vi "Anritsu VNA Get Stimulus.vi"(7 "Anritsu VNA":T1, 8 "error in (no error)":errorcluster, 9 "Channel":i8=1 min=1 max=99 step=1, 11 "VISA Resource Name":refnum<visa-resource-name>) -> (0 "error out":errorcluster, 2 "SP Stimulus":T2={"Use Instrument Settings"=FALSE, "Blank Frequencies"=FALSE, "Sweep Type"=enum."Linear", "Sweep"={"Fstart"=500.0, "Fstop"=1500.0, "Units"=enum."MHz", "Points"=201}, "Power (dBm)"=999.0, "IFBW (Hz)"=-1.0, "Sweep Time (s)"=-1.0, "Calibration"={"State"=FALSE, "String"=""}} {"Sweep Time (s)" format="%.3g"}, 3 "dup VISA Resource Name":refnum<visa-resource-name>)   [LabVIEW 2011]
uses:
  tests/S Parameter/TypeDefs/SP Stimulus Parameters.ctl
  tests/S Parameter/TypeDefs/SP Frequency Units.ctl
  tests/S Parameter/TypeDefs/SP Calibration State.ctl
  TypeDefs/Anritsu VNA Instrument Info.ctl
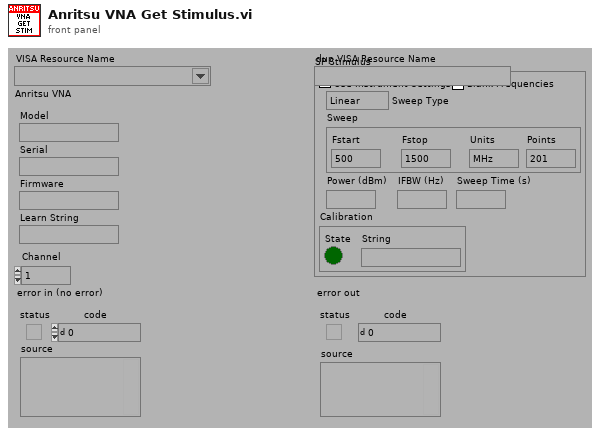
[diagram p1: front panel]
types:
  T1 = typedef "Anritsu VNA Instrument Info.ctl" = cluster{"Model":string, "Serial":string, "Firmware":string, "Learn String":string}
  T2 = typedef "SP Stimulus Parameters.ctl" = cluster{"Use Instrument Settings":bool, "Blank Frequencies":bool, "Sweep Type":enum32{"Linear", "Logarithmic", "List", "Power", "CW"}, "Sweep":cluster{"Fstart":dbl, "Fstop":dbl, "Units":T3, "Points":i32}, "Power (dBm)":dbl, "IFBW (Hz)":dbl, "Sweep Time (s)":dbl, "Calibration":T4}
  T3 = typedef "SP Frequency Units.ctl" = enum16{"Hz", "kHz", "MHz", "GHz", "Points"}
  T4 = typedef "SP Calibration State.ctl" = cluster{"State":bool, "String":string}
  T5 = typedef "Anritsu VNA Sweep Type.ctl" = enum32{"Linear Sweep", "Frequency Sweep", "Power Sweep", "CW Time Sweep", "Discrete Fill", "Time Domain", "Logarithmic Sweep", "Segmented Sweep (Frequency)", "Segmented Sweep (Index)", "MFGC"}
  T6 = enum32{"Linear", "Logarithmic", "List", "Power", "CW"}
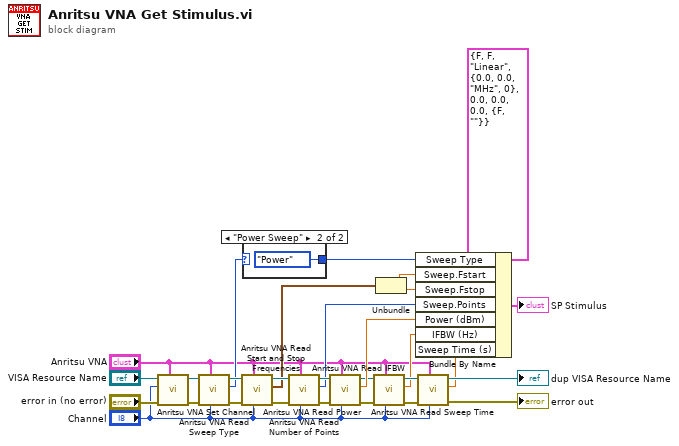
[diagram p0: block diagram]
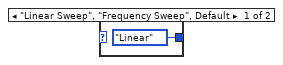
[diagram p2: hidden frame]
diagram:
  n1 = call "Anritsu VNA Set Channel.vi"("Anritsu VNA"="Anritsu VNA", "error in (no error)"="error in (no error)", "Channel"="Channel", "VISA Resource Name"="VISA Resource Name") -> ("error out"=w3:errorcluster, "dup VISA Resource Name"=w4:refnum<visa-resource-name>)  [unwired: 6 out]
  n2 = call "Anritsu VNA Read Sweep Type.vi"("Channel"="Channel", "Anritsu VNA"="Anritsu VNA", "error in (no error)"=w3, "VISA Resource Name"=w4) -> ("error out"=w27:errorcluster, "Sweep Type"=w20:T5, "dup VISA Resource Name"=w26:refnum<visa-resource-name>)  [unwired: 5 out]
  n3 = call "Anritsu VNA Read Start and Stop Frequencies.vi"("Channel"="Channel", "Anritsu VNA"="Anritsu VNA", "error in (no error)"=w27, "VISA Resource Name"=w26) -> ("error out"=w25:errorcluster, "Start/Stop Freqs, MHz"=w8:cluster{"Fstart":dbl, "Fstop":dbl}, "dup VISA Resource Name"=w24:refnum<visa-resource-name>)  [unwired: 5 out]
  n4 = case shown="\"Power Sweep\"" w20 {
    tunnel: [T6."Linear" ("Sweep Type") T6."Power" ("Sweep Type")] -> w7
    frame "Linear Sweep", "Frequency Sweep", Default {
    }
    frame "Power Sweep" {
    }
  }
  n5 = call "Anritsu VNA Read Number of Points.vi"("Channel"="Channel", "Anritsu VNA"="Anritsu VNA", "error in (no error)"=w25, "VISA Resource Name"=w24) -> ("error out"=w22:errorcluster, "Number Points"=w11:i32, "dup VISA Resource Name"=w23:refnum<visa-resource-name>)  [unwired: 5 out]
  n6 = call "Anritsu VNA Read Power.vi"("Channel"="Channel", "Anritsu VNA"="Anritsu VNA", "error in (no error)"=w22, "VISA Resource Name"=w23) -> ("error out"=w14:errorcluster, "Source Power, dBm"=w28:dbl, "dup VISA Resource Name"=w19:refnum<visa-resource-name>)  [unwired: 5 out]
  n7 = call "Anritsu VNA Read IFBW.vi"("Channel"="Channel", "Anritsu VNA"="Anritsu VNA", "error in (no error)"=w14, "VISA Resource Name"=w19) -> ("error out"=w15:errorcluster, "IFBW, Hz"=w12:dbl, "dup VISA Resource Name"=w18:refnum<visa-resource-name>)  [unwired: 5 out]
  n8 = Unbundle(w8) -> ("Fstart"=w9:dbl, "Fstop"=w10:dbl)
  n9 = call "Anritsu VNA Read Sweep Time.vi"("Channel"="Channel", "Anritsu VNA"="Anritsu VNA", "error in (no error)"=w15, "VISA Resource Name"=w18) -> ("error out"=→"error out":errorcluster, "Sweep Time, s"=w13:dbl, "dup VISA Resource Name"=→"dup VISA Resource Name":refnum<visa-resource-name>)  [unwired: 5 out]
  n10 = Bundle By Name(cluster=T2 {"Use Instrument Settings"=FALSE, "Blank Frequencies"=FALSE, "Sweep Type"=enum."Linear", "Sweep"={"Fstart"=0.0, "Fstop"=0.0, "Units"=enum."MHz", "Points"=0}, "Power (dBm)"=0.0, "IFBW (Hz)"=0.0, "Sweep Time (s)"=0.0, "Calibration"={"State"=FALSE, "String"=""}} ("Stimulus"), "Sweep Type"=w7, "Sweep.Fstart"=w9, "Sweep.Fstop"=w10, "Sweep.Points"=w11, "Power (dBm)"=w28, "IFBW (Hz)"=w12, "Sweep Time (s)"=w13) -> (→"SP Stimulus":T2)
